vi "Disconnect.vi"(8 "error in (no error)":errorcluster, 11 "CameraDemo in":refnum<class "Camera.lvclass">) -> (0 "error out":errorcluster, 3 "CameraDemo out":refnum<class "Camera.lvclass">)   [LabVIEW 2020, in "CameraI2COUSB.lvlib" / "Camera.lvclass"]
doc: "Close connection to camera"
uses:
  Camera.lvclass
  Camera.lvclass/Camera.ctl
  CameraDriver/II2COUSB/II2COUSB/II2COUSB.lvclass
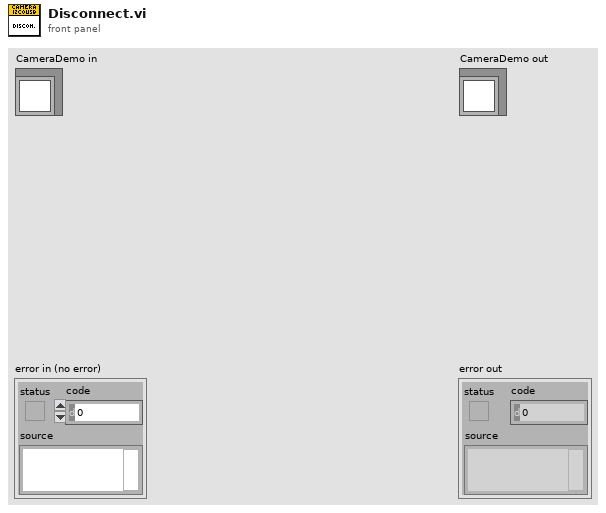
[diagram p1: front panel]
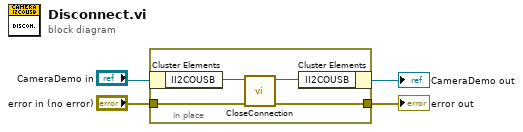
[diagram p0: block diagram]
diagram:
  n1 = in-place {
    in-place-border: "error in (no error)" -> [w6]
    in-place-border: [w5] -> w2
    n2 = in-place-cluster #1("CameraDemo in") -> ("II2COUSB"=w8:refnum<class "II2COUSB.lvclass">)
    n3 = call-dynamic "CloseConnection.vi"("error in (no error)"=w6, "II2COUSB in"=w8) -> ("error out"=w5:errorcluster, "II2COUSB out"=w7:refnum<class "II2COUSB.lvclass">)  [unwired: 7 in, 1 out]
    n4 = in-place-cluster #1("II2COUSB"=w7) -> (→"CameraDemo out":refnum<class "Camera.lvclass">)
  }
  "error out" <- w2
